vi "Evaluate Part 2.vi"() -> ()   [LabVIEW 2020]
uses:
  Measurement/Measurement.lvclass
panel:
  out "sum":i64
  in  "Input":string="0 3 6 9 12 15\n1 3 6 10 15 21\n10 13 16 21 30 45"
  # "1853145127 -> too high"
  # "1853145120 -> Too high"
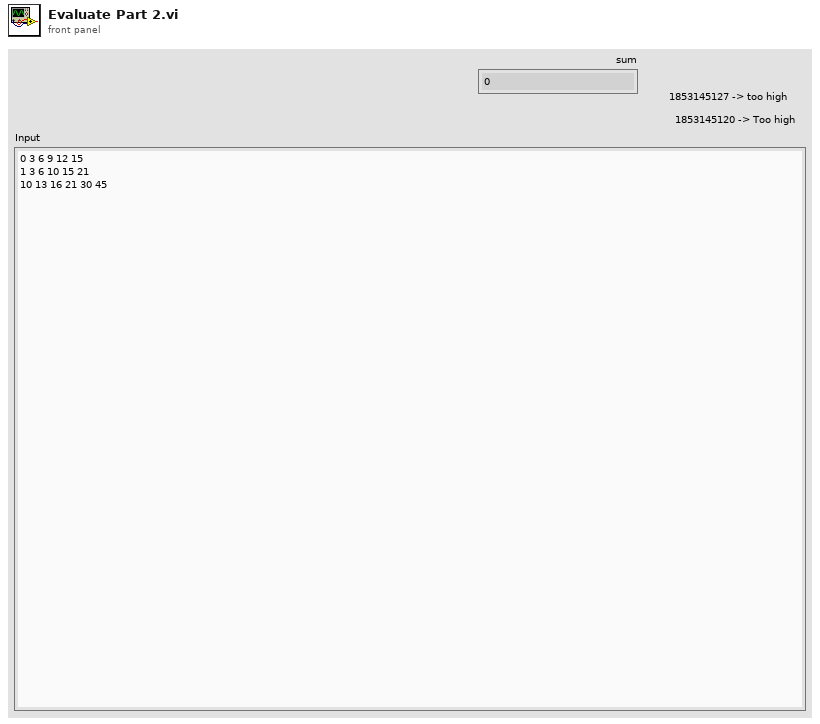
[diagram p1: front panel]
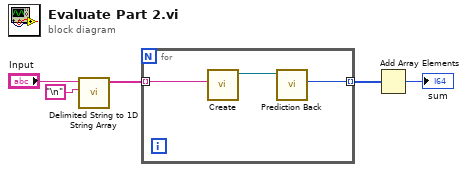
[diagram p0: block diagram]
diagram:
  n1 = call <vilib>:"Delimited String to 1D String Array.vi"("delimiter"="\n", "delimited string"="Input") -> ("string array"=w3:string[])  [unwired: 9 in]
  n2 = for {
    tunnel: w3 -> [w7] mode=indexing
    tunnel: [w6] -> w1 mode=indexing
    n3 = call "Create.vi"("Input"=w7) -> ("Measurement"=w8:refnum<class "Measurement.lvclass">)  [unwired: 9 in, 1 out]
    n4 = call "Prediction Back.vi"("Measurement in"=w8) -> ("Numeric"=w6:i64)  [unwired: 8 in, 2 out]
  }
  n5 = Add Array Elements(numeric array=w1) -> (sum=→"sum":i64)
